vi "detailsCustomer.vi"(0 "reference in":refnum<class "excelFile.lvclass">, 2 "TSR_details":T1={"Company/Institution:"="", "Address:"="", "Department:"="", "City:"="", "Post Code:"="", "Country:"="", "Contact:"="", "Ref:"="", "Issue description:"="", "Actions:"="", "TYPE:"="Repair", "Shipping:"=0, "Discount:"=0, "dataIN"=[], "Device type:"="microQuark", "Serial Number:"="", "PMC number:"="", "Labour Hours:"=0.0, "Service Location:"=FALSE, "start_hour"="", "end_hour"="", "o2_exp_date"="", "GST"=TRUE}, 5 "error in (no error)":errorcluster) -> (14 "reference out":refnum<class "excelFile.lvclass">, 19 "error out":errorcluster)   [LabVIEW 2016, in "excelFile.lvclass"]
uses:
  excelFile.lvclass
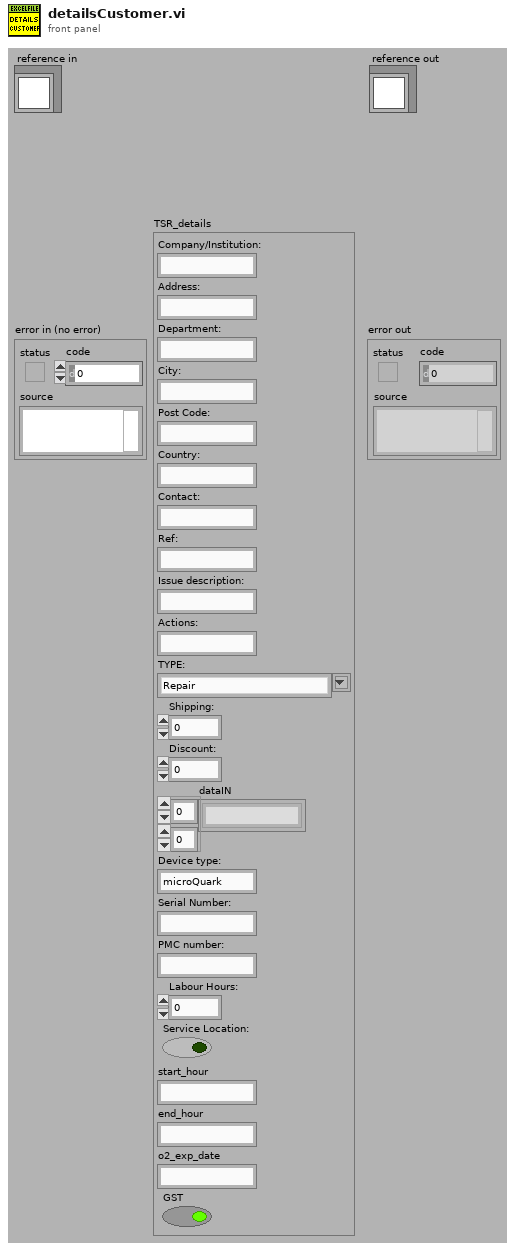
[diagram p1: front panel]
types:
  T1 = cluster{"Company/Institution:":string, "Address:":string, "Department:":string, "City:":string, "Post Code:":string, "Country:":string, "Contact:":string, "Ref:":string, "Issue description:":string, "Actions:":string, "TYPE:":string, "Shipping:":i32, "Discount:":i32, "dataIN":string[][], "Device type:":string, "Serial Number:":string, "PMC number:":string, "Labour Hours:":dbl, "Service Location:":bool, "start_hour":string, "end_hour":string, "o2_exp_date":string, "GST":bool}
  T2 = typedef "excelFile.lvclass/ObjectAttributesRef.ctl" = refnum<data-value>
  T3 = typedef "excelFile.lvclass/ObjectAttributes.ctl" = cluster{"MyAttribute":dbl, "path":string, "Refnum Excel":cluster{"Excel._Application":refnum<k7>, "Workbooks":refnum<k7>, "Open":refnum<k7>}, "data":string[][][], "save":bool, "fileType":T4, "rowsColor":u32[], "python_ref":refnum<class "python.lvclass">, "items_rows":i32[], "excel_range":i32[][], "TSR":cluster{"number":string, "TSR_path":path, "service_path":path, "email_to":string}, "excel_already_opened?":bool, "file_already_opened?":bool, "excel_protected_opened?":bool, "Refnum Cluster Worksheets":cluster{"Excel._Application":refnum<k7>, "Workbooks":refnum<k7>, "Open":refnum<k7>, "Worksheets":refnum<k7>, "Excel._Worksheet":refnum<k7>}, "#_rows_defective":i32, "#_rows_spare":i32}
  T4 = typedef "excelFile.lvclass/fileType.ctl" = enum16{"devices", "items", "partsTracking", "TSR"}
  T5 = cluster{"number":string, "TSR_path":path, "service_path":path, "email_to":string}
  T6 = cluster{"Excel._Application":refnum<k7>, "Workbooks":refnum<k7>, "Open":refnum<k7>}
  T7 = cluster{"Excel._Application":refnum<k7>, "Workbooks":refnum<k7>, "Open":refnum<k7>, "Worksheets":refnum<k7>, "Excel._Worksheet":refnum<k7>}
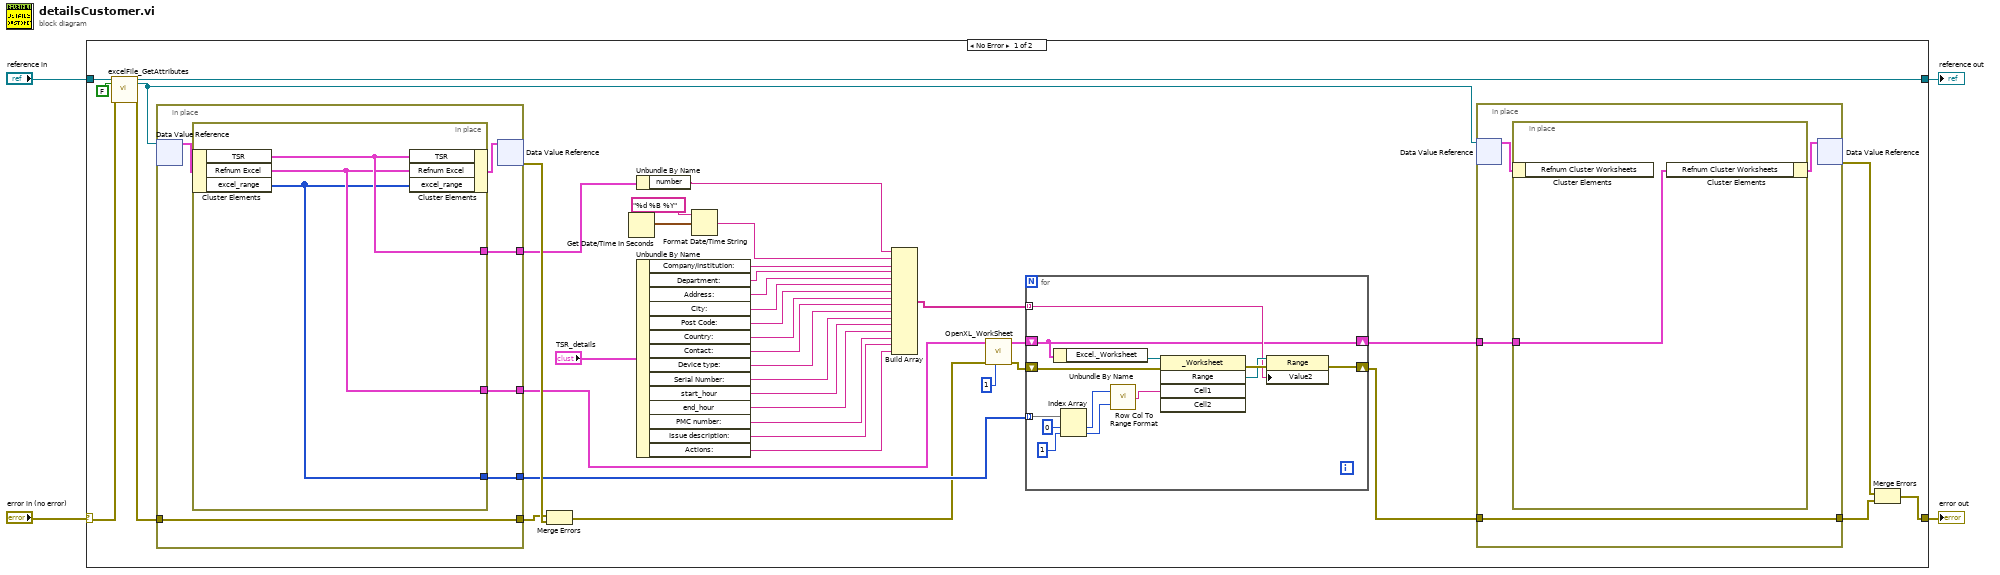
[diagram p0: block diagram]
diagram:
  n1 = case shown="No Error" "error in (no error)" {
    selector: "error in (no error)" -> [w40 w73]
    tunnel: [w6 w73] -> w3
    tunnel: [w38 w72] -> w1
    tunnel: "reference in" -> [w42 w72]
    frame No Error {
      n2 = call "excelFile_GetAttributes.vi"("reference in"=w42, "return data? (T)"=FALSE, "error in (no error)"=w40) -> ("reference out"=w38:refnum<class "excelFile.lvclass">, "attributes ref"=w9:T2, "error out"=w39:errorcluster)  [unwired: 13 in, 1 out]
      n3 = in-place {
        in-place-border: w39 -> [w66]
        in-place-border: [w66] -> w43
        in-place-border: [w65] -> w19
        in-place-border: [w64] -> w18
        in-place-border: [w63] -> w15
        n4 = in-place-dvr #1(w9) -> (w67:T3)  [unwired: 1 out]
        n5 = in-place {
          in-place-border: [w71] -> w65
          in-place-border: [w70] -> w64
          in-place-border: [w69] -> w63
          n6 = in-place-cluster #2(w67) -> ("TSR"=w71:T5, "Refnum Excel"=w70:T6, "excel_range"=w69:i32[][])
          n7 = in-place-cluster #2("TSR"=w71, "Refnum Excel"=w70, "excel_range"=w69) -> (w68:T3)
        }
        n8 = in-place-dvr #1(w68) -> (w44:errorcluster)  [unwired: 1 out]
      }
      n9 = Merge Errors(w43, w44) -> (w12:errorcluster)
      n10 = Get Date/Time In Seconds() -> (seconds since 1Jan1904=w37:timestamp)
      n11 = Unbundle By Name(w19) -> ("number"=w23:string)
      n12 = Unbundle By Name("TSR_details") -> ("Company/Institution:"=w35:string, "Department:"=w34:string, "Address:"=w33:string, "City:"=w32:string, "Post Code:"=w31:string, "Country:"=w30:string, "Contact:"=w29:string, "Device type:"=w28:string, "Serial Number:"=w27:string, "start_hour"=w21:string, "end_hour"=w20:string, "PMC number:"=w26:string, "Issue description:"=w25:string, "Actions:"=w24:string)
      n13 = Format Date/Time String(time format string (%c)="%d %B %Y", seconds (now)=w37) -> (date/time string=w22:string)  [unwired: 1 in]
      n14 = Build Array(w23, w22, w35, w34, w33, w32, w31, w30, w29, w28, w27, w21, w20, w26, w25, w24) -> (w16:string[])
      n15 = call <userlib>:"OpenXL_WorkSheet.vi"("Sheet"=1, "error in (no error)"=w12, "Refnum Cluster In"=w18) -> ("error out"=w14:errorcluster, "Refnum Cluster Out"=w17:T7)  [unwired: 7 in]
      n16 = for {
        shift-right: [w51] -> w11
        shift-left: w14 -> [w53]
        shift-right: [w50] -> w10
        shift-left: w17 -> [w50]
        tunnel: w15 -> [w58] mode=indexing
        tunnel: w16 -> [w52] mode=indexing
        n17 = Unbundle By Name(w50) -> ("Excel._Worksheet"=w59:refnum<k7>)
        n18 = Index Array(array=w58, index #1=0 ("index"), index #2=1 ("index")) -> (element #1=w55:i32, element #2=w54:i32)
        n19 = call <userlib>:"Row Col To Range Format.vi"("Column"=w54, "Row"=w55) -> ("Output String"=w62:string)
        n20 = invoke class="_Worksheet" method="Range"(reference=w59, error in=w53, "Cell1"=w62) -> (error out=w61:errorcluster, "Range"=w60:refnum<k7>)  [unwired: 2 in, 3 out]
        n21 = property class="Range"(reference=w60, error in=w61, "Value2"=w52) -> (error out=w51:errorcluster)  [unwired: 1 out]
      }
      n22 = in-place {
        in-place-border: w11 -> [w46]
        in-place-border: [w46] -> w8
        in-place-border: w10 -> [w45]
        n23 = in-place-dvr #3(w9) -> (w47:T3)  [unwired: 1 out]
        n24 = in-place {
          in-place-border: w45 -> [w49]
          n25 = in-place-cluster #4(w47) -> ()  [unwired: 1 out]
          n26 = in-place-cluster #4("Refnum Cluster Worksheets"=w49) -> (w48:T3)
        }
        n27 = in-place-dvr #3(w48) -> (w7:errorcluster)  [unwired: 1 out]
      }
      n28 = Merge Errors(w7, w8) -> (w6:errorcluster)
    }
    frame Error {
    }
  }
  "error out" <- w3
  "reference out" <- w1
